vi "Update Attribute Tree.vi"(4 "error in":errorcluster, 5 "Flush Tree?":bool, 6 "Tree Control In":refnum<vi>, 7 "Camera Name In":T1 caption="Session In") -> (0 "error out":errorcluster, 2 "Tree Control Out":refnum<vi>, 3 "Session Out":T1)   [LabVIEW 2012]
doc: "The Update Attribute Tree subVI, enumerates the attributes available for the camera and populates the Attribute Tree control with the attribute list."
uses:
  <vilib>/userDefined/High Color/IMAQdx.ctl
  <vilib>/vision/driver/NI_Vision_Acquisition_Software.lvlib
  <resource>/objmgr/imaqdx.rc
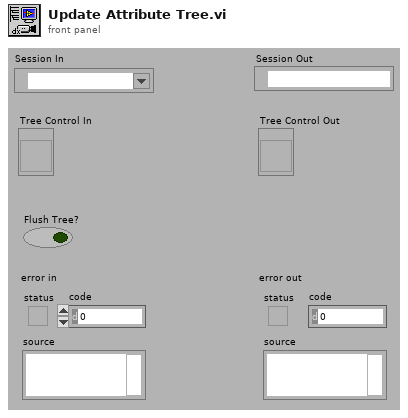
[diagram p1: front panel]
types:
  T1 = typedef "IMAQdx.ctl" = refnum<k21>
  T2 = typedef "NI_Vision_Acquisition_Software.lvlib/IMAQdx Attribute Type.ctl" = enum32{"U32", "I64", "DBL", "String", "Enum", "Bool", "Command"}
  T3 = cluster{"Attribute Type":T2, "Readable":bool, "Writable":bool, "Attribute Name":string}[]
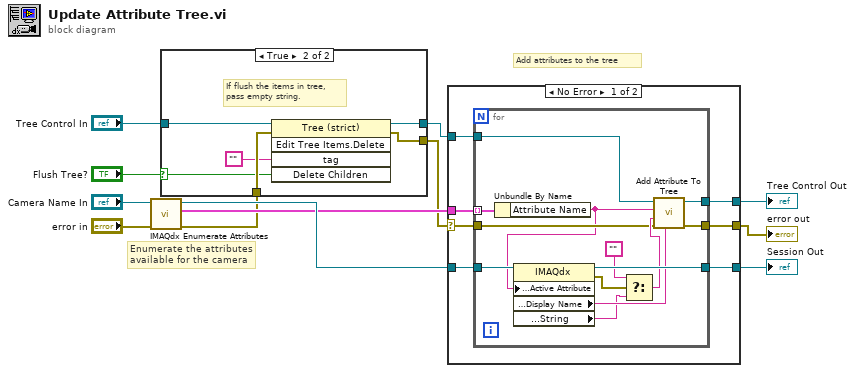
[diagram p0: block diagram]
diagram:
  # "Add attributes to the tree"
  # "Enumerate the attributes \navailable for the camera"
  n1 = call <vilib>:"IMAQdx Enumerate Attributes.vi"("error in"="error in", "Session In"="Camera Name In") -> ("error out"=w4:errorcluster, "Attribute Information Array"=w11:T3, "Session Out"=w12:T1)  [unwired: 2 in, 5 out]
  n2 = case shown="True" "Flush Tree?" {
    selector: "Flush Tree?" -> [_ w15]
    tunnel: [w14 w20] -> w6
    tunnel: [w13 w19] -> w5
    tunnel: w4 -> [w13 w18]
    tunnel: "Tree Control In" -> [w14 w16]
    frame False {
    }
    frame True {
      # "If flush the items in tree,\npass empty string."
      n3 = invoke class="Tree (strict)" method="Edit Tree Items.Delete"(reference=w16, error in=w18, "tag"="", "Delete Children"=w15) -> (reference out=w20:refnum<vi>, error out=w19:errorcluster)  [unwired: 1 in, 3 out]
    }
  }
  n4 = case shown="No Error" w5 {
    selector: w5 -> [w25 w43]
    tunnel: w11 -> [w27 _]
    tunnel: w6 -> [w26 w41]
    tunnel: w12 -> [w24 w42]
    tunnel: [w23 w43] -> w3
    tunnel: [w22 w42] -> w8
    tunnel: [w21 w41] -> w7
    frame No Error {
      n5 = for {
        tunnel: w27 -> [w40] mode=indexing
        tunnel: w26 -> [w36]
        tunnel: w25 -> [w32]
        tunnel: w24 -> [w39]
        tunnel: [w38] -> w23
        tunnel: [w37] -> w22
        tunnel: [w31] -> w21
        n6 = Unbundle By Name(w40) -> ("Attribute Name"=w30:string)
        n7 = property class="IMAQdx"(reference=w39, "Camera Attributes:Active Attribute"=w30) -> (reference out=w37:T1, error out=w35:errorcluster, "Camera Attributes:Display Name"=w29:string, "Camera Attributes:Value:String"=w28:string)  [unwired: 1 in]
        n8 = Select(t="", s=w35, f=w28) -> (s? t:f=w34:string)
        n9 = call "Add Attribute To Tree.vi"("Display Name"=w29, "error in"=w32, "Value"=w34, "Attribute Name"=w30, "Attribute Table In"=w36) -> ("error out"=w38:errorcluster, "Attribute Table Out"=w31:refnum<vi>)  [unwired: 5 out]
      }
    }
    frame Error {
    }
  }
  "error out" <- w3
  "Session Out" <- w8
  "Tree Control Out" <- w7
